vi "Calc Battery.vi"(9 "Batt 280":dbl, 10 "Batt310":dbl, 11 "AD":dbl) -> (3 "Batt Volt":dbl)   [LabVIEW 2015]
uses:
  <vilib>/Analysis/baseanly.llb/Mean (DBL).vi
  <vilib>/Analysis/NI_AALBase.lvlib
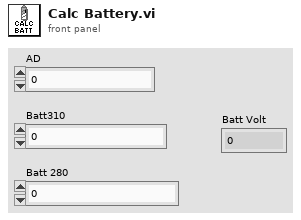
[diagram p1: front panel]
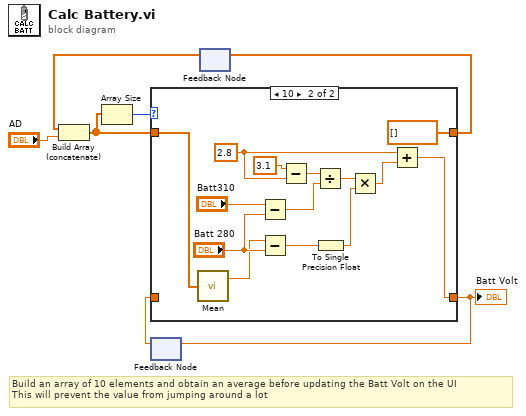
[diagram p0: block diagram]
diagram:
  # "Build an array of 10 elements and obtain an average before updating the Batt Volt on the UI\nThis will prevent the value from jumping around a lot"
  n1 = feedback #1() -> (w1:dbl)  [unwired: 1 in]
  n2 = feedback #2() -> (w6:dbl[])  [unwired: 1 in]
  n3 = Build Array (concatenate)(w6, "AD") -> (w4:dbl[])
  n4 = Array Size(array=w4) -> (size(s)=w5:i32)
  n5 = case shown="10" w5 {
    tunnel: w4 -> [w9 w13]
    tunnel: [w9 dbl[] []] -> w3
    tunnel: [w8 w10] -> w2
    tunnel: w1 -> [w8 _]
    frame Default {
    }
    frame 10 {
      w17 = 2.8
      n6 = call-poly <vilib>:"Mean.vi"("X"=w13) -> ("mean"=w12:dbl)  [unwired: 1 out]
      n7 = Subtract(x="Batt310", y="Batt 280") -> (x-y=w19:dbl)
      n8 = Subtract(x=w12, y="Batt 280") -> (x-y=w15:dbl)
      n9 = Subtract(x=3.1, y=w17) -> (x-y=w20:dbl)
      n10 = Divide(x=w20, y=w19) -> (x/y=w16:dbl)
      n11 = To Single Precision Float(number=w15) -> (single precision float=w14:sgl)
      n12 = Multiply(x=w16, y=w14) -> (x*y=w18:dbl)
      n13 = Add(x=w17, y=w18) -> (x+y=w10:dbl)
    }
  }
  "Batt Volt" <- w2
  n14 = feedback-in #1(w2) -> ()
  n15 = feedback-in #2(w3) -> ()
